vi "Simple Add.vi"(10 "y":dbl, 11 "x":dbl) -> (3 "x+y":dbl)   [LabVIEW 2018]
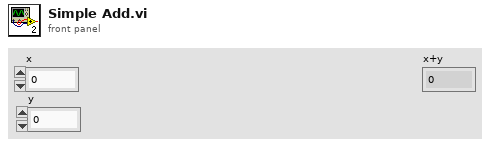
[diagram p1: front panel]
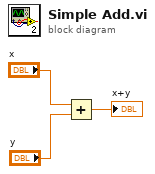
[diagram p0: block diagram]
diagram:
  n1 = Add(x="x", y="y") -> (x+y=→"x+y":dbl)
